vi "Hella CAN Diesel.vi"(0 "Command (kPa)":u16, 11 "Error In":errorcluster) -> (15 "Error Out":errorcluster)   [LabVIEW 2019]
uses:
  CAN Mode.ctl
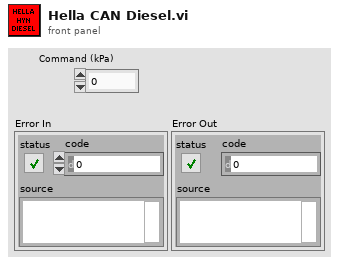
[diagram p1: front panel]
types:
  T1 = typedef "CAN Mode.ctl" = enum16{"Init", "Read", "Write", "Close"}
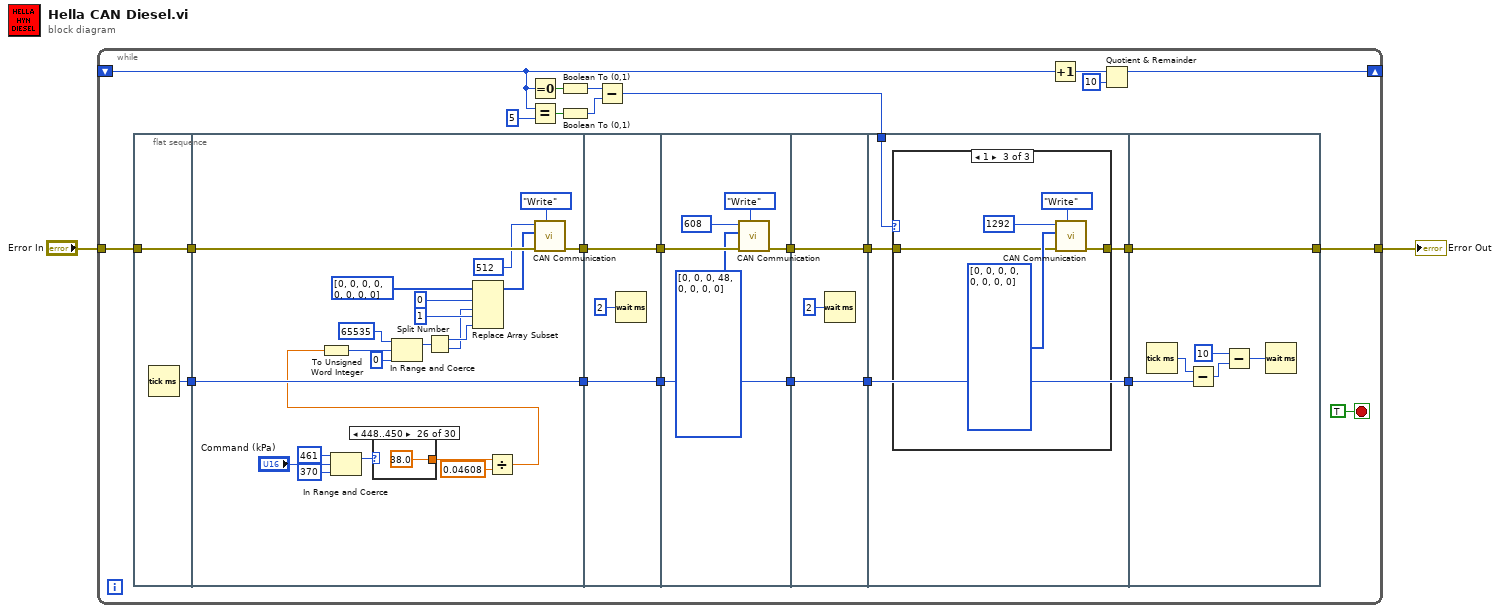
[diagram p0: block diagram]
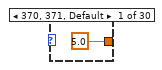
[diagram p2: hidden frame]
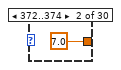
[diagram p3: hidden frame]
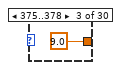
[diagram p4: hidden frame]
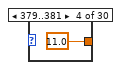
[diagram p5: hidden frame]
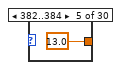
[diagram p6: hidden frame]
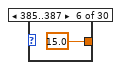
[diagram p7: hidden frame]
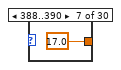
[diagram p8: hidden frame]
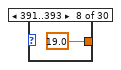
[diagram p9: hidden frame]
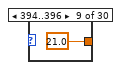
[diagram p10: hidden frame]
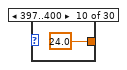
[diagram p11: hidden frame]
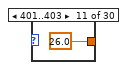
[diagram p12: hidden frame]
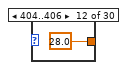
[diagram p13: hidden frame]
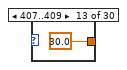
[diagram p14: hidden frame]
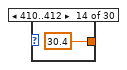
[diagram p15: hidden frame]
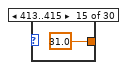
[diagram p16: hidden frame]
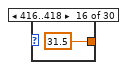
[diagram p17: hidden frame]
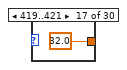
[diagram p18: hidden frame]
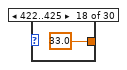
[diagram p19: hidden frame]
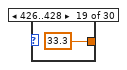
[diagram p20: hidden frame]
diagram:
  n1 = while {
    tunnel: "Error In" -> [w27]
    shift-right: [w14] -> _
    shift-left: _ -> [w13]
    tunnel: [w4] -> w1
    stop <- TRUE stop-if-true
    n2 = flat-sequence {
      tunnel: w27 -> [w29]
      tunnel: [w29] -> w26
      tunnel: [w28] -> w6
      tunnel: w26 -> [w51]
      tunnel: [w50] -> w25
      tunnel: [w49] -> w7
      tunnel: w6 -> [w49]
      tunnel: w25 -> [w83]
      tunnel: [w83] -> w24
      tunnel: [w82] -> w8
      tunnel: w7 -> [w82]
      tunnel: w24 -> [w90]
      tunnel: [w89] -> w22
      tunnel: [w88] -> w9
      tunnel: w8 -> [w88]
      tunnel: [w92] -> w23
      tunnel: w22 -> [w92]
      tunnel: [w91] -> w10
      tunnel: w9 -> [w91]
      tunnel: w23 -> [w97]
      tunnel: w12 -> [w96]
      tunnel: [w95] -> w11
      tunnel: w10 -> [w95]
      tunnel: [w94] -> w3
      tunnel: w11 -> [w121]
      tunnel: [w116] -> w4
      tunnel: w3 -> [w116]
      frame #0 {
        n3 = Tick Count (ms)() -> (millisecond timer value=w28:u32)
      }
      frame #1 {
        n4 = In Range and Coerce(upper limit=u16 461, x="Command (kPa)", lower limit=u16 370) -> (coerced(x)=w33:u16)  [unwired: 1 out]
        n5 = case shown="448..450" w33 {
          tunnel: [5.0 ("Command (kPa)") 7.0 ("Command (kPa)") 9.0 ("Command (kPa)") 11.0 ("Command (kPa)") 13.0 ("Command (kPa)") 15.0 ("Command (kPa)") 17.0 ("Command (kPa)") 19.0 ("Command (kPa)") 21.0 ("Command (kPa)") 24.0 ("Command (kPa)") 26.0 ("Command (kPa)") 28.0 ("Command (kPa)") 30.0 ("Command (kPa)") 30.4 ("Command (kPa)") 31.0 ("Command (kPa)") 31.5 ("Command (kPa)") 32.0 ("Command (kPa)") 33.0 ("Command (kPa)") 33.3 ("Command (kPa)") 34.0 ("Command (kPa)") 34.7 ("Command (kPa)") 35.0 ("Command (kPa)") 36.0 ("Command (kPa)") 36.5 ("Command (kPa)") 37.0 ("Command (kPa)") 38.0 ("Command (kPa)") 38.3 ("Command (kPa)") 39.0 ("Command (kPa)") 39.7 ("Command (kPa)") 40.0 ("Command (kPa)")] -> w32
          frame 370, 371, Default {
          }
          frame 372..374 {
          }
          frame 375..378 {
          }
          frame 379..381 {
          }
          frame 382..384 {
          }
          frame 385..387 {
          }
          frame 388..390 {
          }
          frame 391..393 {
          }
          frame 394..396 {
          }
          frame 397..400 {
          }
          frame 401..403 {
          }
          frame 404..406 {
          }
          frame 407..409 {
          }
          frame 410..412 {
          }
          frame 413..415 {
          }
          frame 416..418 {
          }
          frame 419..421 {
          }
          frame 422..425 {
          }
          frame 426..428 {
          }
          frame 429..431 {
          }
          frame 432..434 {
          }
          frame 435..437 {
          }
          frame 438..440 {
          }
          frame 441..443 {
          }
          frame 444..447 {
          }
          frame 448..450 {
          }
          frame 451..453 {
          }
          frame 454..456 {
          }
          frame 457..459 {
          }
          frame 460, 461 {
          }
        }
        n6 = Divide(x=w32, y=0.04608) -> (x/y=w30:dbl)
        n7 = To Unsigned Word Integer(number=w30) -> (unsigned 16bit integer=w43:u16)
        n8 = In Range and Coerce(upper limit=u16 65535, x=w43, lower limit=u16 0) -> (coerced(x)=w40:u16)  [unwired: 1 out]
        n9 = Split Number(x=w40) -> (hi(x)=w38:u8, lo(x)=w37:u8)
        n10 = Replace Array Subset(array=u8[] [0, 0, 0, 0, 0, 0, 0, 0] ("Data Array (Hex) Bytes  0 -> 7"), new element #1=w37, index #1=0 ("index"), new element #2=w38, index #2=1 ("index")) -> (w47:u8[])
        n11 = call "CAN Communication.vi"("CAN Mode"=CAN_Mode."Write", "Error IN"=w51, "Message"=w47, "Arbitration ID"=u32 512) -> ("Error OUT"=w50:errorcluster)  [unwired: 6 in, 1 out]
      }
      frame #2 {
        n12 = Wait (ms)(milliseconds to wait=u32 2) -> ()  [unwired: 1 out]
      }
      frame #3 {
        n13 = call "CAN Communication.vi"("CAN Mode"=CAN_Mode."Write", "Error IN"=w90, "Message"=u8[] [0, 0, 0, 48, 0, 0, 0, 0] ("Data frame to 0x260"), "Arbitration ID"=u32 608 ("CAN Addres to Xmit\nSpeed CMD (Hex) 2")) -> ("Error OUT"=w89:errorcluster)  [unwired: 6 in, 1 out]
      }
      frame #4 {
        n14 = Wait (ms)(milliseconds to wait=u32 2) -> ()  [unwired: 1 out]
      }
      frame #5 {
        n15 = case shown="1" w96 {
          tunnel: w97 -> [w102 w104 w112]
          tunnel: [w101 w103 w111] -> w94
          frame -1 {
            n16 = call "CAN Communication.vi"("CAN Mode"=CAN_Mode."Write", "Error IN"=w102, "Message"=u8[] [0, 0, 0, 134, 0, 0, 0, 93] ("Data frame to 0x545"), "Arbitration ID"=u32 1349) -> ("Error OUT"=w101:errorcluster)  [unwired: 6 in, 1 out]
          }
          frame Default {
            n17 = case shown="Error" w104 {
              selector: w104 -> [w105 _]
              tunnel: [w105 w106] -> w103
              frame No Error {
              }
              frame Error {
                n18 = call "CAN Communication.vi"("CAN Mode"=CAN_Mode."Close", "Error IN"=errorcluster {"status"=FALSE, "code"=0, "source"=""}) -> ("Error OUT"=w108:errorcluster)  [unwired: 8 in, 1 out]
                n19 = call "CAN Communication.vi"("CAN Mode"=CAN_Mode."Init", "Error IN"=w108) -> ("Error OUT"=w106:errorcluster)  [unwired: 8 in, 1 out]
              }
            }
          }
          frame 1 {
            n20 = call "CAN Communication.vi"("CAN Mode"=CAN_Mode."Write", "Error IN"=w112, "Message"=u8[] [0, 0, 0, 0, 0, 0, 0, 0] ("Data frame to 0x50C"), "Arbitration ID"=u32 1292) -> ("Error OUT"=w111:errorcluster)  [unwired: 6 in, 1 out]
          }
        }
      }
      frame #6 {
        n21 = Tick Count (ms)() -> (millisecond timer value=w120:u32)
        n22 = Subtract(x=w120, y=w121) -> (x-y=w119:u32)
        n23 = Subtract(x=u32 10, y=w119) -> (x-y=w117:u32)
        n24 = Wait (ms)(milliseconds to wait=w117) -> ()  [unwired: 1 out]
      }
    }
    n25 = Equal To 0?(x=w13) -> (x = 0?=w18:bool)
    n26 = Equal?(x=w13, y=u32 5) -> (x = y?=w19:bool)
    n27 = Boolean To (0,1)(Boolean=w18) -> (0, 1=w20:i16)
    n28 = Boolean To (0,1)(Boolean=w19) -> (0, 1=w21:i16)
    n29 = Subtract(x=w20, y=w21) -> (x-y=w12:i16)
    n30 = Increment(x=w13) -> (x+1=w15:u32)
    n31 = Quotient & Remainder(x=w15, y=u32 10) -> (x-y*floor(x/y)=w14:u32)  [unwired: 1 out]
  }
  "Error Out" <- w1
